vi "多参数数据插入.vi"(8 "error in (no error)":errorcluster caption="错误输入（无错误）", 9 "编号":string, 10 "columns enable":T1, 11 "data in":T2) -> (0 "error out":errorcluster)   [LabVIEW 2016, in "斯坦道多参数.lvlib"]
uses:
  <vilib>/addons/database/Auxilliary.llb/DB Tools Column Info.ctl
  <vilib>/addons/database/Auxilliary.llb/DB Tools DataTypes.ctl
  <vilib>/addons/database/NI_Database_API.lvlib
  WxMessage/wxpusher.lvlib
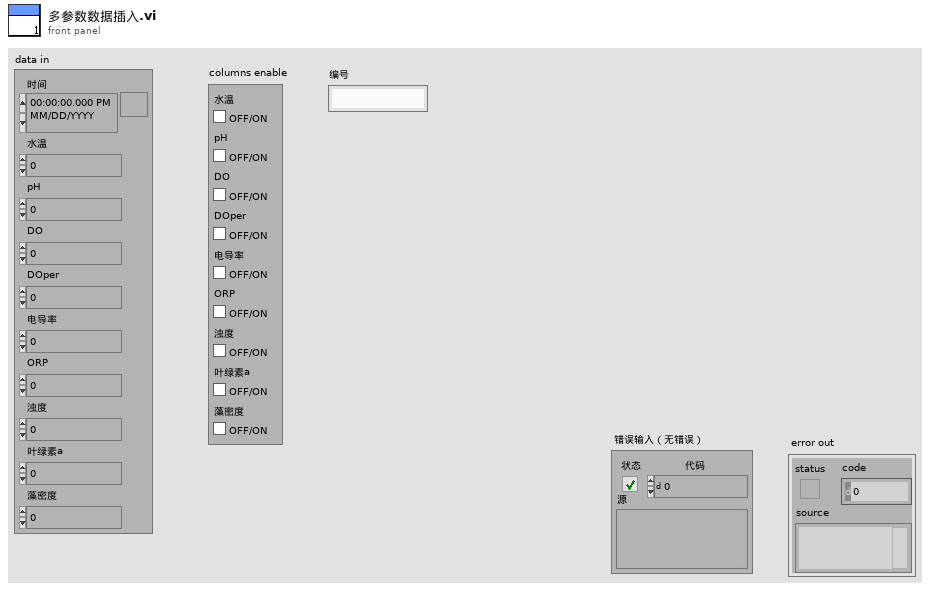
[diagram p1: front panel]
types:
  T1 = cluster{"水温":bool, "pH":bool, "DO":bool, "DOper":bool, "电导率":bool, "ORP":bool, "浊度":bool, "叶绿素a":bool, "藻密度":bool}
  T2 = cluster{"时间":timestamp, "水温":dbl, "pH":dbl, "DO":dbl, "DOper":dbl, "电导率":dbl, "ORP":dbl, "浊度":dbl, "叶绿素a":dbl, "藻密度":dbl}
  T3 = typedef "NI_Database_API.lvlib/DB Tools Column Info.ctl" = cluster{"column name":string, "data type":T4, "size":i32, "allow null?":bool}
  T4 = typedef "NI_Database_API.lvlib/DB Tools DataTypes.ctl" = enum16{"String", "Long (I32)", "Single (SGL)", "Double (DBL)", "Date/Time", "Binary"}
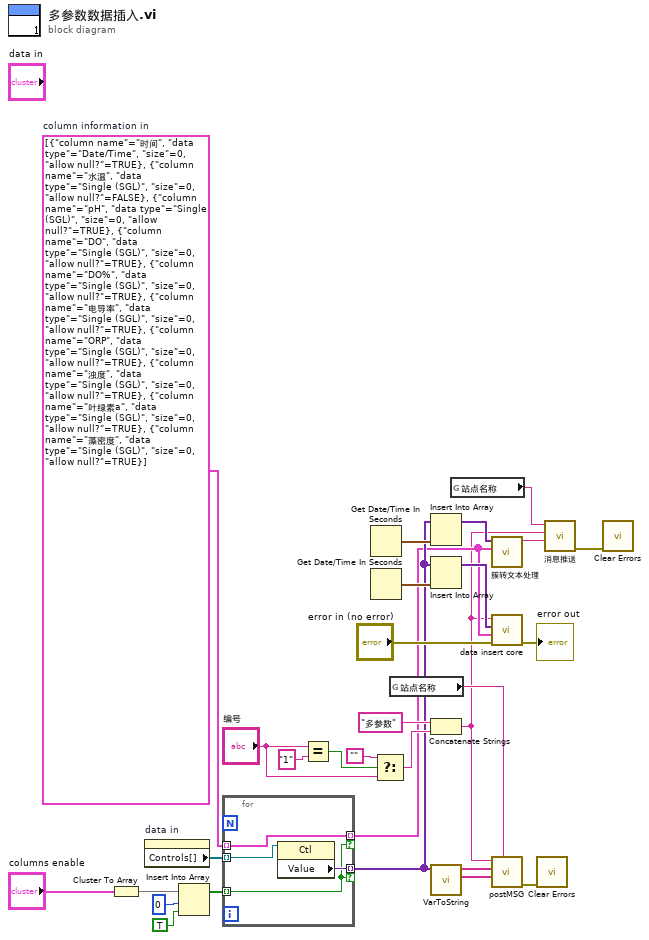
[diagram p0: block diagram]
diagram:
  w19 = T3[] [{"column name"="时间", "data type"=enum."Date/Time", "size"=0, "allow null?"=TRUE}, {"column name"="水温", "data type"=enum."Single (SGL)", "size"=0, "allow null?"=FALSE}, {"column name"="pH", "data type"=enum."Single (SGL)", "size"=0, "allow null?"=TRUE}, {"column name"="DO", "data type"=enum."Single (SGL)", "size"=0, "allow null?"=TRUE}, {"column name"="DO%", "data type"=enum."Single (SGL)", "size"=0, "allow null?"=TRUE}, {"column name"="电导率", "data type"=enum."Single (SGL)", "size"=0, "allow null?"=TRUE}, {"column name"="ORP", "data type"=enum."Single (SGL)", "size"=0, "allow null?"=TRUE}, {"column name"="浊度", "data type"=enum."Single (SGL)", "size"=0, "allow null?"=TRUE}, {"column name"="叶绿素a", "data type"=enum."Single (SGL)", "size"=0, "allow null?"=TRUE}, {"column name"="藻密度", "data type"=enum."Single (SGL)", "size"=0, "allow null?"=TRUE}]  # column information in
  n1 = Cluster To Array(cluster="columns enable") -> (array=w16:bool[])
  n2 = property on="data in" class="Clust (严格)"() -> ("Controls[]"=w22:refnum<vi>[])  [unwired: 2 in, 2 out]
  n3 = Insert Into Array(array=w16, index=0 ("索引"), new element=TRUE ("新元素/子数组")) -> (w17:bool[])
  n4 = for {
    tunnel: w22 -> [w33] mode=indexing
    tunnel: [w32] -> w6 mode=indexing if=w30
    tunnel: w19 -> [w31] mode=indexing
    tunnel: [w31] -> w5 mode=indexing if=w30
    tunnel: w17 -> [w30] mode=indexing
    n5 = property class="Ctl"(reference=w33) -> ("Value"=w32:variant)  [unwired: 1 in, 2 out]
  }
  n6 = Equal?(x="编号", y="1") -> (x = y?=w26:bool)
  n7 = Get Date/Time In Seconds() -> (seconds since 1Jan1904=w13:timestamp)
  n8 = Get Date/Time In Seconds() -> (seconds since 1Jan1904=w21:timestamp)
  n9 = Select(t="", s=w26, f="编号") -> (s? t:f=w23:string)
  n10 = global read "系统设置全局变量.vi" "站点名称"() -> (w9:string)
  n11 = Insert Into Array(array=w6, new element=w13) -> (w10:variant[])  [unwired: 1 in]
  n12 = Insert Into Array(array=w6, new element=w21) -> (w20:variant[])  [unwired: 1 in]
  n13 = Concatenate Strings("多参数" ("字符串"), w23) -> (w4:string)
  n14 = call "VarToString.vi"("数组"=w6) -> ("data"=w7:string[], "columns"=w8:string[])  [unwired: 9 in]
  n15 = global read "系统设置全局变量.vi" "站点名称"() -> (w11:string)
  n16 = call "簇转文本处理.vi"("column information"=w5, "data"=w10) -> ("output"=w12:string)  [unwired: 9 in]
  n17 = call "data insert core.vi"("error in (no error)"="error in (no error)", "column information"=w5, "data"=w20, "table"=w4) -> ("error out"=→"error out":errorcluster)  [unwired: 7 in]
  n18 = call "postMSG.vi"("station"=w9, "data"=w7, "columns"=w8, "table"=w4) -> ("error out"=w2:errorcluster)  [unwired: 7 in]
  n19 = call <vilib>:"Clear Errors.vi"("error in (no error)"=w2) -> ()  [unwired: 5 in, 2 out]
  n20 = call "消息推送.vi"("数据内容"=w12, "参数"=w4, "站点"=w11) -> ("error out"=w1:errorcluster)  [unwired: 8 in]
  n21 = call <vilib>:"Clear Errors.vi"("error in (no error)"=w1) -> ()  [unwired: 5 in, 2 out]
